vi "On Change Camera Focus.vi"(6 "Updated At":u32, 8 "error in (no error)":errorcluster, 10 "Focus Value":i32, 11 "App in":refnum<class "App.lvclass">) -> (0 "error out":errorcluster, 3 "App out":refnum<class "App.lvclass">)   [LabVIEW 2020, in "AR Example.lvlib" / "App.lvclass"]
uses:
  App.lvclass
  App.lvclass/App.ctl
  0449e33a-8b8a-4cd6-a04c-8828b9bf9353.vi
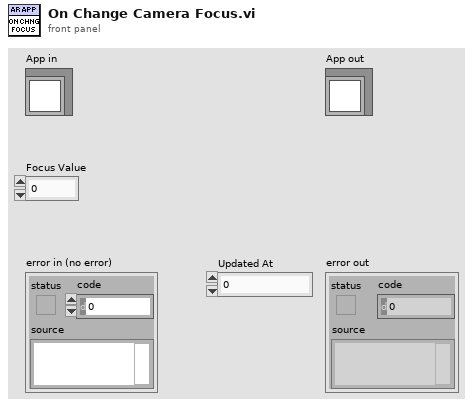
[diagram p1: front panel]
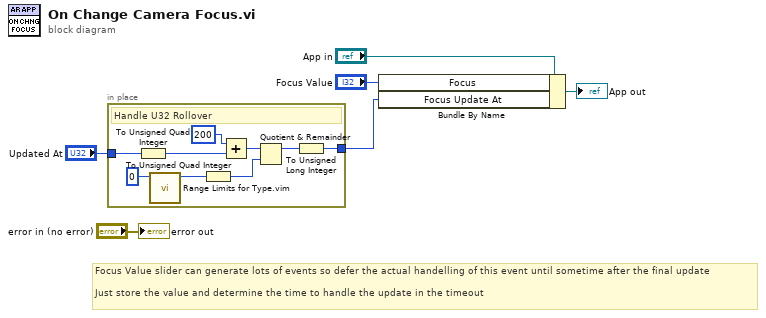
[diagram p0: block diagram]
diagram:
  # "Focus Value slider can generate lots of events so defer the actual handelling of this event until sometime after the final update\n\nJust store the value and determine the time to handle the update in the timeout"
  n1 = in-place {
    in-place-border: "Updated At" -> [w15]
    in-place-border: [w7] -> w1
    # "Handle U32 Rollover"
    n2 = To Unsigned Quad Integer(1:w15) -> (0:w13:u64)
    n3 = call "Range Limits for Type.vim"("type"=u32 0) -> ("maximum value for type"=w10:u32)  [unwired: 9 in, 1 out]
    n4 = To Unsigned Quad Integer(1:w10) -> (0:w9:u64)
    n5 = Add(x=u64 200, y=w13) -> (x+y=w12:u64)
    n6 = Quotient & Remainder(x=w12, y=w9) -> (x-y*floor(x/y)=w8:u64)  [unwired: 1 out]
    n7 = To Unsigned Long Integer(number=w8) -> (unsigned 32bit integer=w7:u32)
  }
  n8 = Bundle By Name(cluster="App in", "Focus"="Focus Value", "Focus Update At"=w1) -> (→"App out":refnum<class "App.lvclass">)
  "error out" <- "error in (no error)"
